vi "arb_scale.vi"(10 "wf":dbl[](array[numeric])) -> (2 "data":i16[](array[numeric]))   [LabVIEW 2017, in "wf.lvlib"]
uses:
  wf.lvlib
panel:
  out "Waveform Graph":i16[](graph)
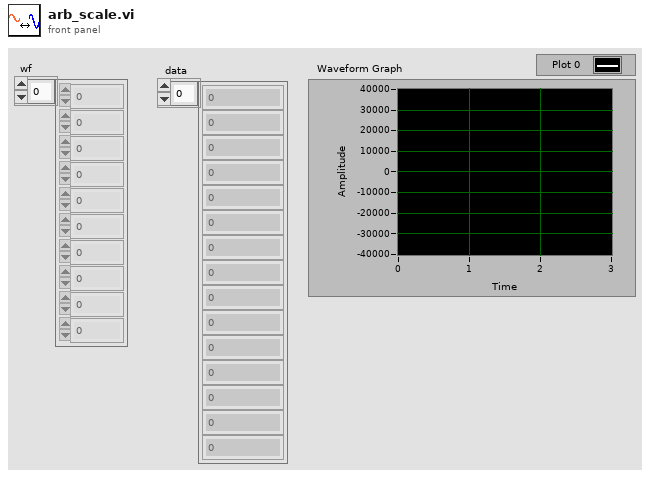
[diagram p1: front panel]
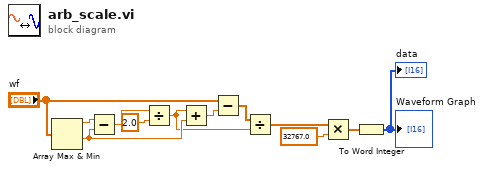
[diagram p0: block diagram]
diagram:
  n1 = Array Max & Min(array="wf") -> (max value=w11:dbl, min value=w10:dbl)  [unwired: 2 out]
  n2 = Subtract(x=w11, y=w10) -> (x-y=w6:dbl)
  n3 = Divide(x=w6, y=2.0) -> (x/y=w2:dbl)
  n4 = Add(x=w2, y=w10) -> (x+y=w4:dbl)
  n5 = Subtract(x="wf", y=w4) -> (x-y=w3:dbl[])
  n6 = Divide(x=w3, y=w2) -> (x/y=w8:dbl[])
  n7 = Multiply(x=w8, y=32767.0) -> (x*y=w12:dbl[])
  n8 = To Word Integer(number=w12) -> (16bit integer=→"data" →"Waveform Graph":i16[])
